vi "Player Info.vi"(11 "Sentinel in":refnum<class "AntFarm_MB.lvclass">) -> (0 "Defeat Speech":string, 1 "Victory Speech":string, 2 "Name":string, 3 "Sentinel out":refnum<class "AntFarm_MB.lvclass">)   [LabVIEW 2016, in "AntFarm_MB.lvclass"]
uses:
  AntFarm_MB.lvclass
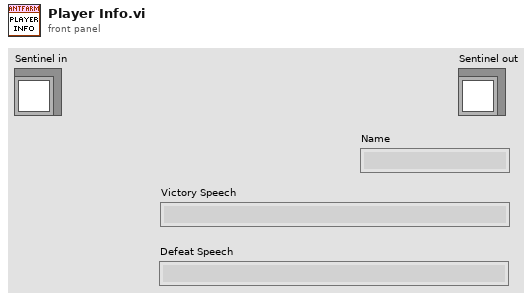
[diagram p1: front panel]
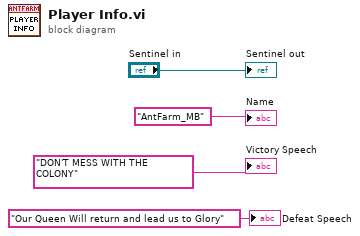
[diagram p0: block diagram]
diagram:
  "Sentinel out" <- "Sentinel in"
  "Name" <- "AntFarm_MB"
  "Victory Speech" <- "DON'T MESS WITH THE COLONY"
  "Defeat Speech" <- "Our Queen Will return and lead us to Glory" ("Defeat Speech")
